vi "TestInitializeDefaultPolicy_PublishOK.vi"(8 "error in (no error)":errorcluster, 11 "TestCase in":refnum<class "TestSubscriptionPolicy.lvclass">) -> (0 "error out":errorcluster, 3 "TestCase out":refnum<class "TestSubscriptionPolicy.lvclass">)   [LabVIEW 2015, in "TestSubscriptionPolicy.lvclass"]
uses:
  TestSubscriptionPolicy.lvclass
  Framework/IMediator/ISubscriptionPolicy/ISubscriptionPolicy.lvclass
  Framework/Transport/QueueTransport/QueueTransport.lvclass
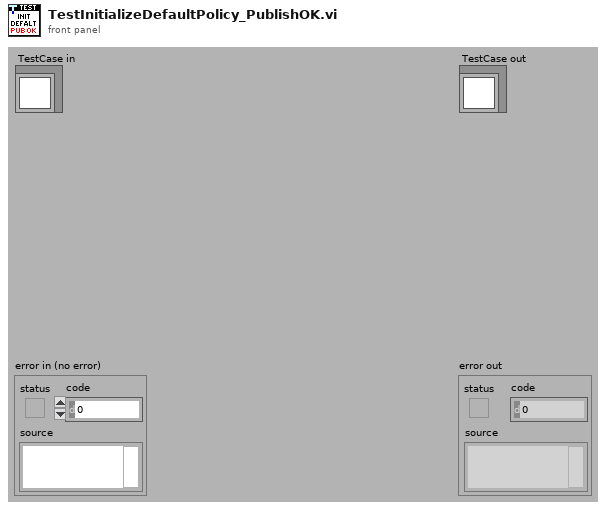
[diagram p1: front panel]
types:
  T1 = typedef "IMediator.lvlib/ISubscriptionPolicy.lvclass/ISubscriptionPolicy Reference.ctl" = refnum<data-value>
  T2 = cluster{"Data":variant, "Publication Time":timestamp}
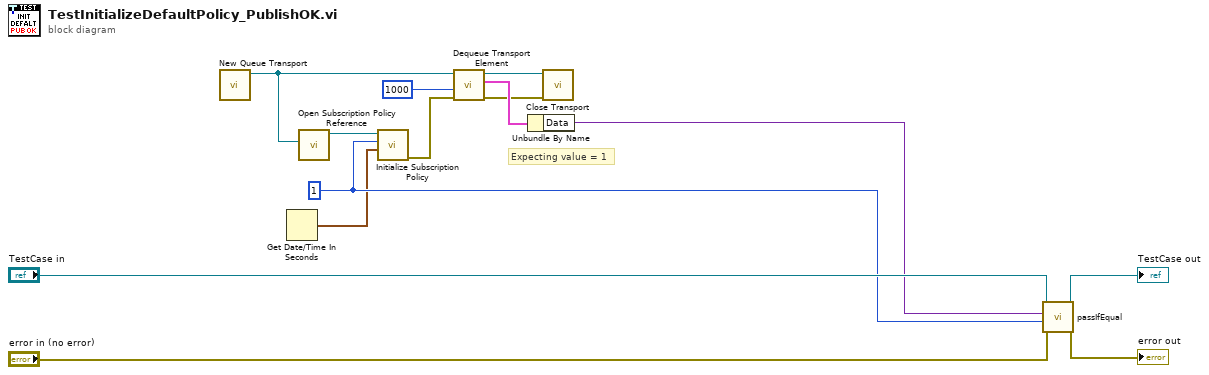
[diagram p0: block diagram]
diagram:
  w4 = 1
  # "Expecting value = 1"
  n1 = call "New Queue Transport.vi"() -> ("QueueTransport Out"=w9:refnum<class "QueueTransport.lvclass">)  [unwired: 10 in, 1 out]
  n2 = Get Date/Time In Seconds() -> (seconds since 1Jan1904=w3:timestamp)
  n3 = call "Open Subscription Policy Reference.vi"("Transport"=w9) -> ("Subscription Policy"=w10:T1)  [unwired: 9 in, 1 out]
  n4 = call "Initialize Subscription Policy.vi"("Last Publish Time"=w3, "Last Topic Value"=w4, "Subscription Policy"=w10) -> ("Error Out (Do Not Subscribe?)"=w8:errorcluster)  [unwired: 8 in]
  n5 = call "Dequeue Transport Element.vi"("error in (no error)"=w8, "Timeout In ms (-1)"=1000, "QueueTransport in"=w9) -> ("error out"=w1:errorcluster, "Element"=w6:T2, "QueueTransport out"=w2:refnum<class "QueueTransport.lvclass">)  [unwired: 5 in, 1 out]
  n6 = Unbundle By Name(w6) -> ("Data"=w5:variant)
  n7 = call-dynamic "Close Transport.vi"("error in (no error)"=w1, "QueueTransport in"=w2) -> ()  [unwired: 9 in, 1 out]
  n8 = call-dynamic "passIfEqual.vi"("error in (no error)"="error in (no error)", "y"=w4, "x"=w5, "TestCase in"="TestCase in") -> ("error out"=→"error out":errorcluster, "TestCase out"=→"TestCase out":refnum<class "TestSubscriptionPolicy.lvclass">)  [unwired: 6 in]
